vi "Initialize XNET Tree.vi"(4 "Info?":refnum<vi>, 6 "Node Ptr":u64 format="%.0x", 8 "error in":errorcluster, 9 "XNET Cluster":refnum<k21>, 10 "XNET Database":refnum<k21>, 11 "Tree":refnum<vi>) -> (0 "error out":errorcluster, 1 "Parent":string, 2 "XNET Cluster Out":refnum<k21>, 3 "Tree Out":refnum<vi>)   [LabVIEW 2019, in "J1939 Addon System Explorer.lvlib"]
uses:
  J1939 Addon System Explorer.lvlib
  Types/CAN Frame Filter.ctl
  Addon Shared/SubVIs/Constants.vi
  <resource>/objmgr/xnet.rc
  <vilib>/NI VeriStand/Custom Device API/Custom Device API.lvlib
  Addon Shared/J1939 Addon Shared.lvlib
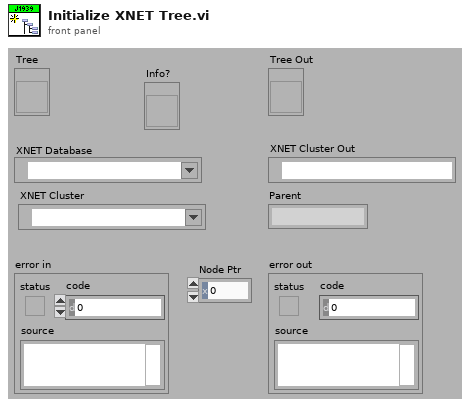
[diagram p1: front panel]
types:
  T1 = typedef "J1939 Addon System Explorer.lvlib/CAN Frame Filter.ctl" = enum16{"Cyclic Data", "Event Data", "Cyclic/Event", "All"}
  T2 = typedef "Custom Device API.lvlib/Custom Device Item Info.ctl" = cluster{"Name":string, "Is Channel":bool, "GUID":string, "Is Waveform":bool}
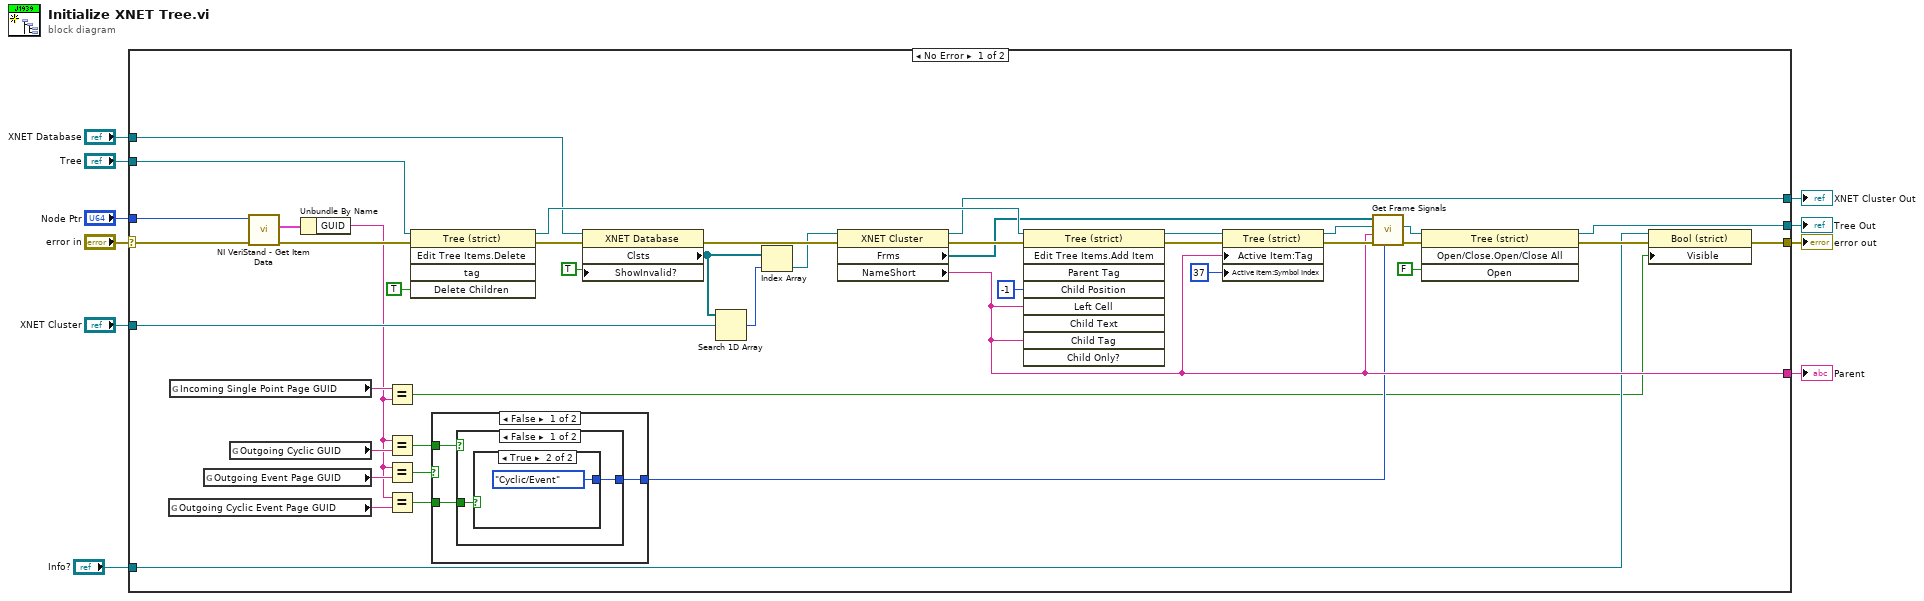
[diagram p0: block diagram]
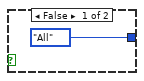
[diagram p2: hidden frame]
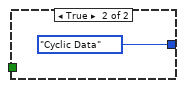
[diagram p3: hidden frame]
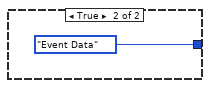
[diagram p4: hidden frame]
diagram:
  n1 = case shown="No Error" "error in" {
    selector: "error in" -> [w27 w64]
    tunnel: "Tree" -> [w51 w63]
    tunnel: [w17 w64] -> w9
    tunnel: "XNET Database" -> [w36 _]
    tunnel: [w39 w63] -> w6
    tunnel: [w41 w62] -> w5
    tunnel: "XNET Cluster" -> [w32 w62]
    tunnel: [w28 _] -> w3
    tunnel: "Node Ptr" -> [w25 _]
    tunnel: "Info?" -> [w16 _]
    frame No Error {
      n2 = global read "Constants.vi" "Outgoing Cyclic Event Page GUID"() -> (w13:string)
      n3 = global read "Constants.vi" "Incoming Single Point Page GUID"() -> (w15:string)
      n4 = global read "Constants.vi" "Outgoing Event Page GUID"() -> (w22:string)
      n5 = global read "Constants.vi" "Outgoing Cyclic GUID"() -> (w23:string)
      n6 = call <vilib>:"NI VeriStand - Get Item Data.vi"("error in (no error)"=w27, "Item Ref in"=w25) -> ("error out"=w26:errorcluster, "Item Info"=w24:T2)  [unwired: 6 in, 2 out]
      n7 = Unbundle By Name(w24) -> ("GUID"=w12:string)
      n8 = Equal?(x=w15, y=w12) -> (x = y?=w14:bool)
      n9 = Equal?(x=w12, y=w23) -> (x = y?=w20:bool)
      n10 = Equal?(x=w12, y=w22) -> (x = y?=w21:bool)
      n11 = Equal?(x=w12, y=w13) -> (x = y?=w11:bool)
      n12 = invoke on="Invoke Node" class="Tree (strict)" method="Edit Tree Items.Delete"(reference=w51, error in=w26, "Delete Children"=TRUE ("Delete Children?")) -> (reference out=w52:refnum<vi>, error out=w34:errorcluster)  [unwired: 2 in, 3 out]
      n13 = case shown="False" w21 {
        tunnel: w20 -> [w55 _]
        tunnel: [w54 CAN_Frame_Filter."Event Data" ("CAN:Timing Type")] -> w19
        tunnel: w11 -> [w53 _]
        frame False {
          n14 = case shown="False" w55 {
            tunnel: [w57 CAN_Frame_Filter."Cyclic Data" ("CAN:Timing Type")] -> w54
            tunnel: w53 -> [w56 _]
            frame False {
              n15 = case shown="True" w56 {
                tunnel: [CAN_Frame_Filter."All" ("CAN:Timing Type") CAN_Frame_Filter."Cyclic/Event" ("CAN:Timing Type")] -> w57
                frame False {
                }
                frame True {
                }
              }
            }
            frame True {
            }
          }
        }
        frame True {
        }
      }
      n16 = property class="XNET Database"(reference=w36, error in=w34, "ShowInvalid?"=TRUE ("Show Invalid From Open?")) -> (error out=w33:errorcluster, "Clsts"=w30:refnum<k21>[])  [unwired: 1 out]
      n17 = Search 1D Array(1D array=w30, element=w32) -> (index of element=w31:i32)  [unwired: 1 in]
      n18 = Index Array(array=w30, index=w31) -> (element=w29:refnum<k21>)
      n19 = property class="XNET Cluster"(reference=w29, error in=w33) -> (reference out=w41:refnum<k21>, error out=w43:errorcluster, "Frms"=w42:refnum<k21>[], "NameShort"=w28:string)
      n20 = invoke on="Invoke Node" class="Tree (strict)" method="Edit Tree Items.Add Item"(reference=w52, error in=w43, "Child Position"=-1, "Left Cell"=w28, "Child Tag"=w28) -> (reference out=w46:refnum<vi>, error out=w45:errorcluster)  [unwired: 4 in, 7 out]
      n21 = property class="Tree (strict)"(reference=w46, error in=w45, "Active Item:Tag"=w28, "Active Item:Symbol Index"=37) -> (reference out=w47:refnum<vi>, error out=w48:errorcluster)
      n22 = call "Get Frame Signals.vi"("CAN:Frame Type"=w19, "error in"=w48, "Parent Tag"=w28, "Tree Reference"=w47, "Frms"=w42) -> ("error out"=w38:errorcluster, "Tree Reference Out"=w37:refnum<vi>)  [unwired: 5 in]
      n23 = invoke on="Invoke Node" class="Tree (strict)" method="Open/Close.Open/Close All"(reference=w37, error in=w38, "Open"=FALSE ("Open?")) -> (reference out=w39:refnum<vi>, error out=w18:errorcluster)  [unwired: 1 in, 2 out]
      n24 = property class="Bool (strict)"(reference=w16, error in=w18, "Visible"=w14) -> (error out=w17:errorcluster)  [unwired: 1 out]
    }
    frame Error {
    }
  }
  "error out" <- w9
  "Tree Out" <- w6
  "XNET Cluster Out" <- w5
  "Parent" <- w3
